vi "R3_Control.vi"() -> ()   [LabVIEW 2016]
uses:
  R3 Reactor Status v1.ctl
  R3 pH Manual Control.ctl
  R3 Pump Manual Control.ctl
  R3Variables.lvlib
panel:
  in  "SBR Timing":T1={"AR feeding"=0.0, "AR Decant"=0.0, "Anoxic feeding (min)"=90.0, "Anaerobic Time (min)"=110.0, "Anaerobic feeding (min)"=5.0, "Anoxic Time (min)"=0.0, "Aerobic Time (min) "=60.0, "Settle (min)"=20.0, "Decant (min)"=3.0}
  in  "R3 Pumps Manual Control":T2
  in  "Reactor 3 pH Control":T3
  out "R3 Reactor Status":T4 {"DO (mg/L)" format="%#_3g"; "pH" format="%#_3g"}
  out "Elapsed Time":dbl
  out "pH and DO":cluster{"pH":dbl, "DO (mg/L)":dbl}(graph)
  out "DO Intercept":dbl
  out "DO Slope":dbl
  out "pH Intercept":dbl
  out "pH Slope":dbl
  in  "pH Control":T5={" pH Set Point"=7.5, " pH Tolerance"=0.1, "Reaction Time (s)"=15.0, "Pump On Time (s)"=3.0}
  in  "Pumps Manual Control":bool
  in  "pH Manual Control":bool
  in  "DO Calibrate":bool
  in  "pH Calibrate":bool
  # "On: Manual Mode\nOff: SBR Mode"
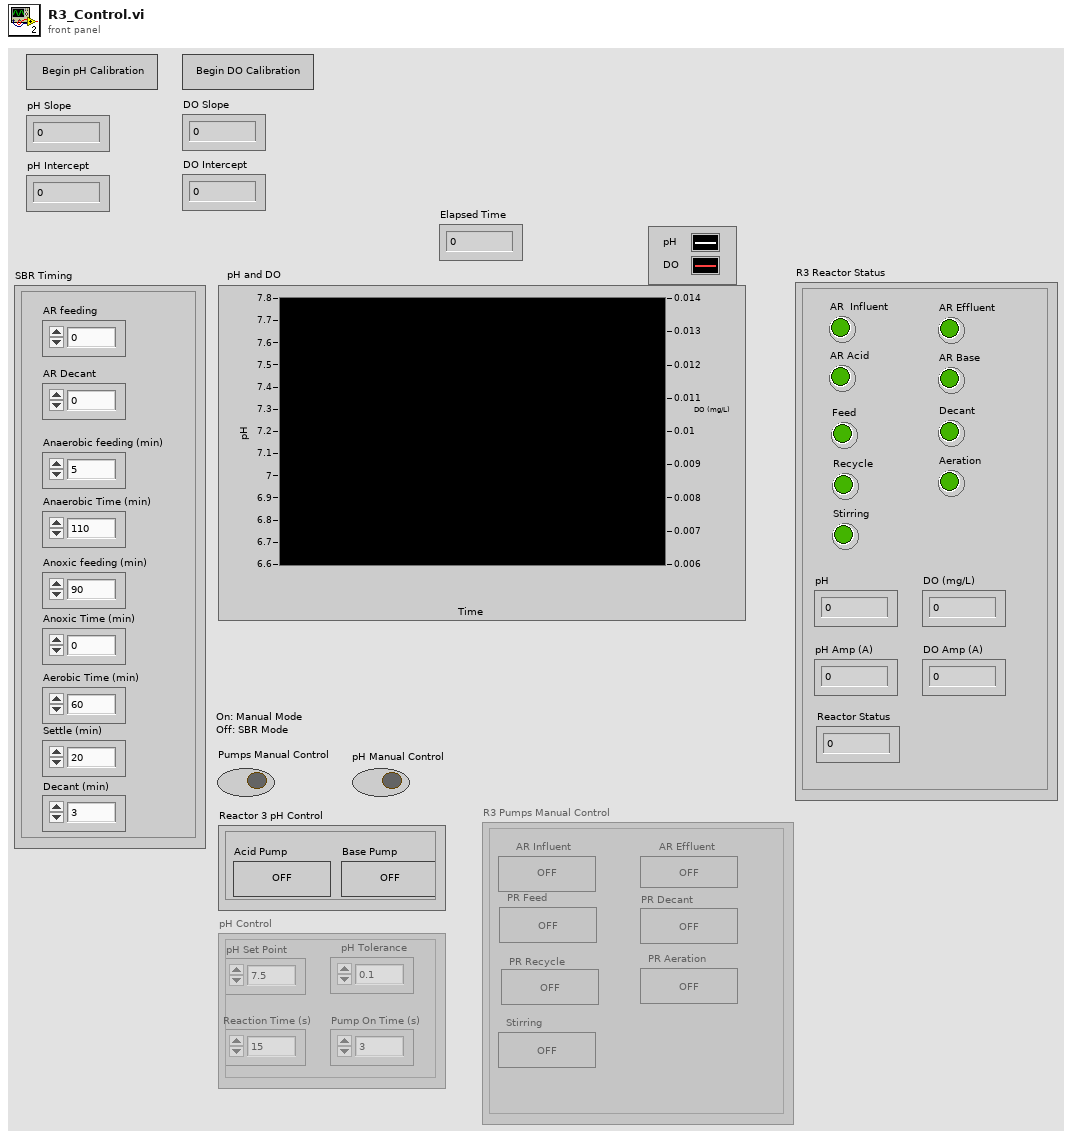
[diagram p1: front panel]
types:
  T1 = cluster{"AR feeding":dbl, "AR Decant":dbl, "Anoxic feeding (min)":dbl, "Anaerobic Time (min)":dbl, "Anaerobic feeding (min)":dbl, "Anoxic Time (min)":dbl, "Aerobic Time (min) ":dbl, "Settle (min)":dbl, "Decant (min)":dbl}
  T2 = cluster{"AR Influent":bool, "AR Effluent":bool, "PR Feed":bool, "PR Decant":bool, "PR Recycle":bool, "PR Aeration":bool, "Stirring":bool}
  T3 = typedef "R3Variables.lvlib/R3 pH Manual Control.ctl" = cluster{"Acid Pump":bool, "Base Pump":bool}
  T4 = typedef "R3Variables.lvlib/R3 Reactor Status v1.ctl" = cluster{"AR  Influent":bool, "AR Effluent":bool, "AR Acid":bool, "AR Base":bool, "Feed":bool, "Aeration":bool, "Decant":bool, "pH":dbl, "DO (mg/L)":dbl, "pH Amp (A)":dbl, "DO Amp (A)":dbl, "Recycle":bool, "Stirring":bool, "Reactor Status":dbl}
  T5 = cluster{" pH Set Point":dbl, " pH Tolerance":dbl, "Reaction Time (s)":dbl, "Pump On Time (s)":dbl}
  T6 = enum8{"Enabled", "Disabled", "Disabled and Grayed Out"}
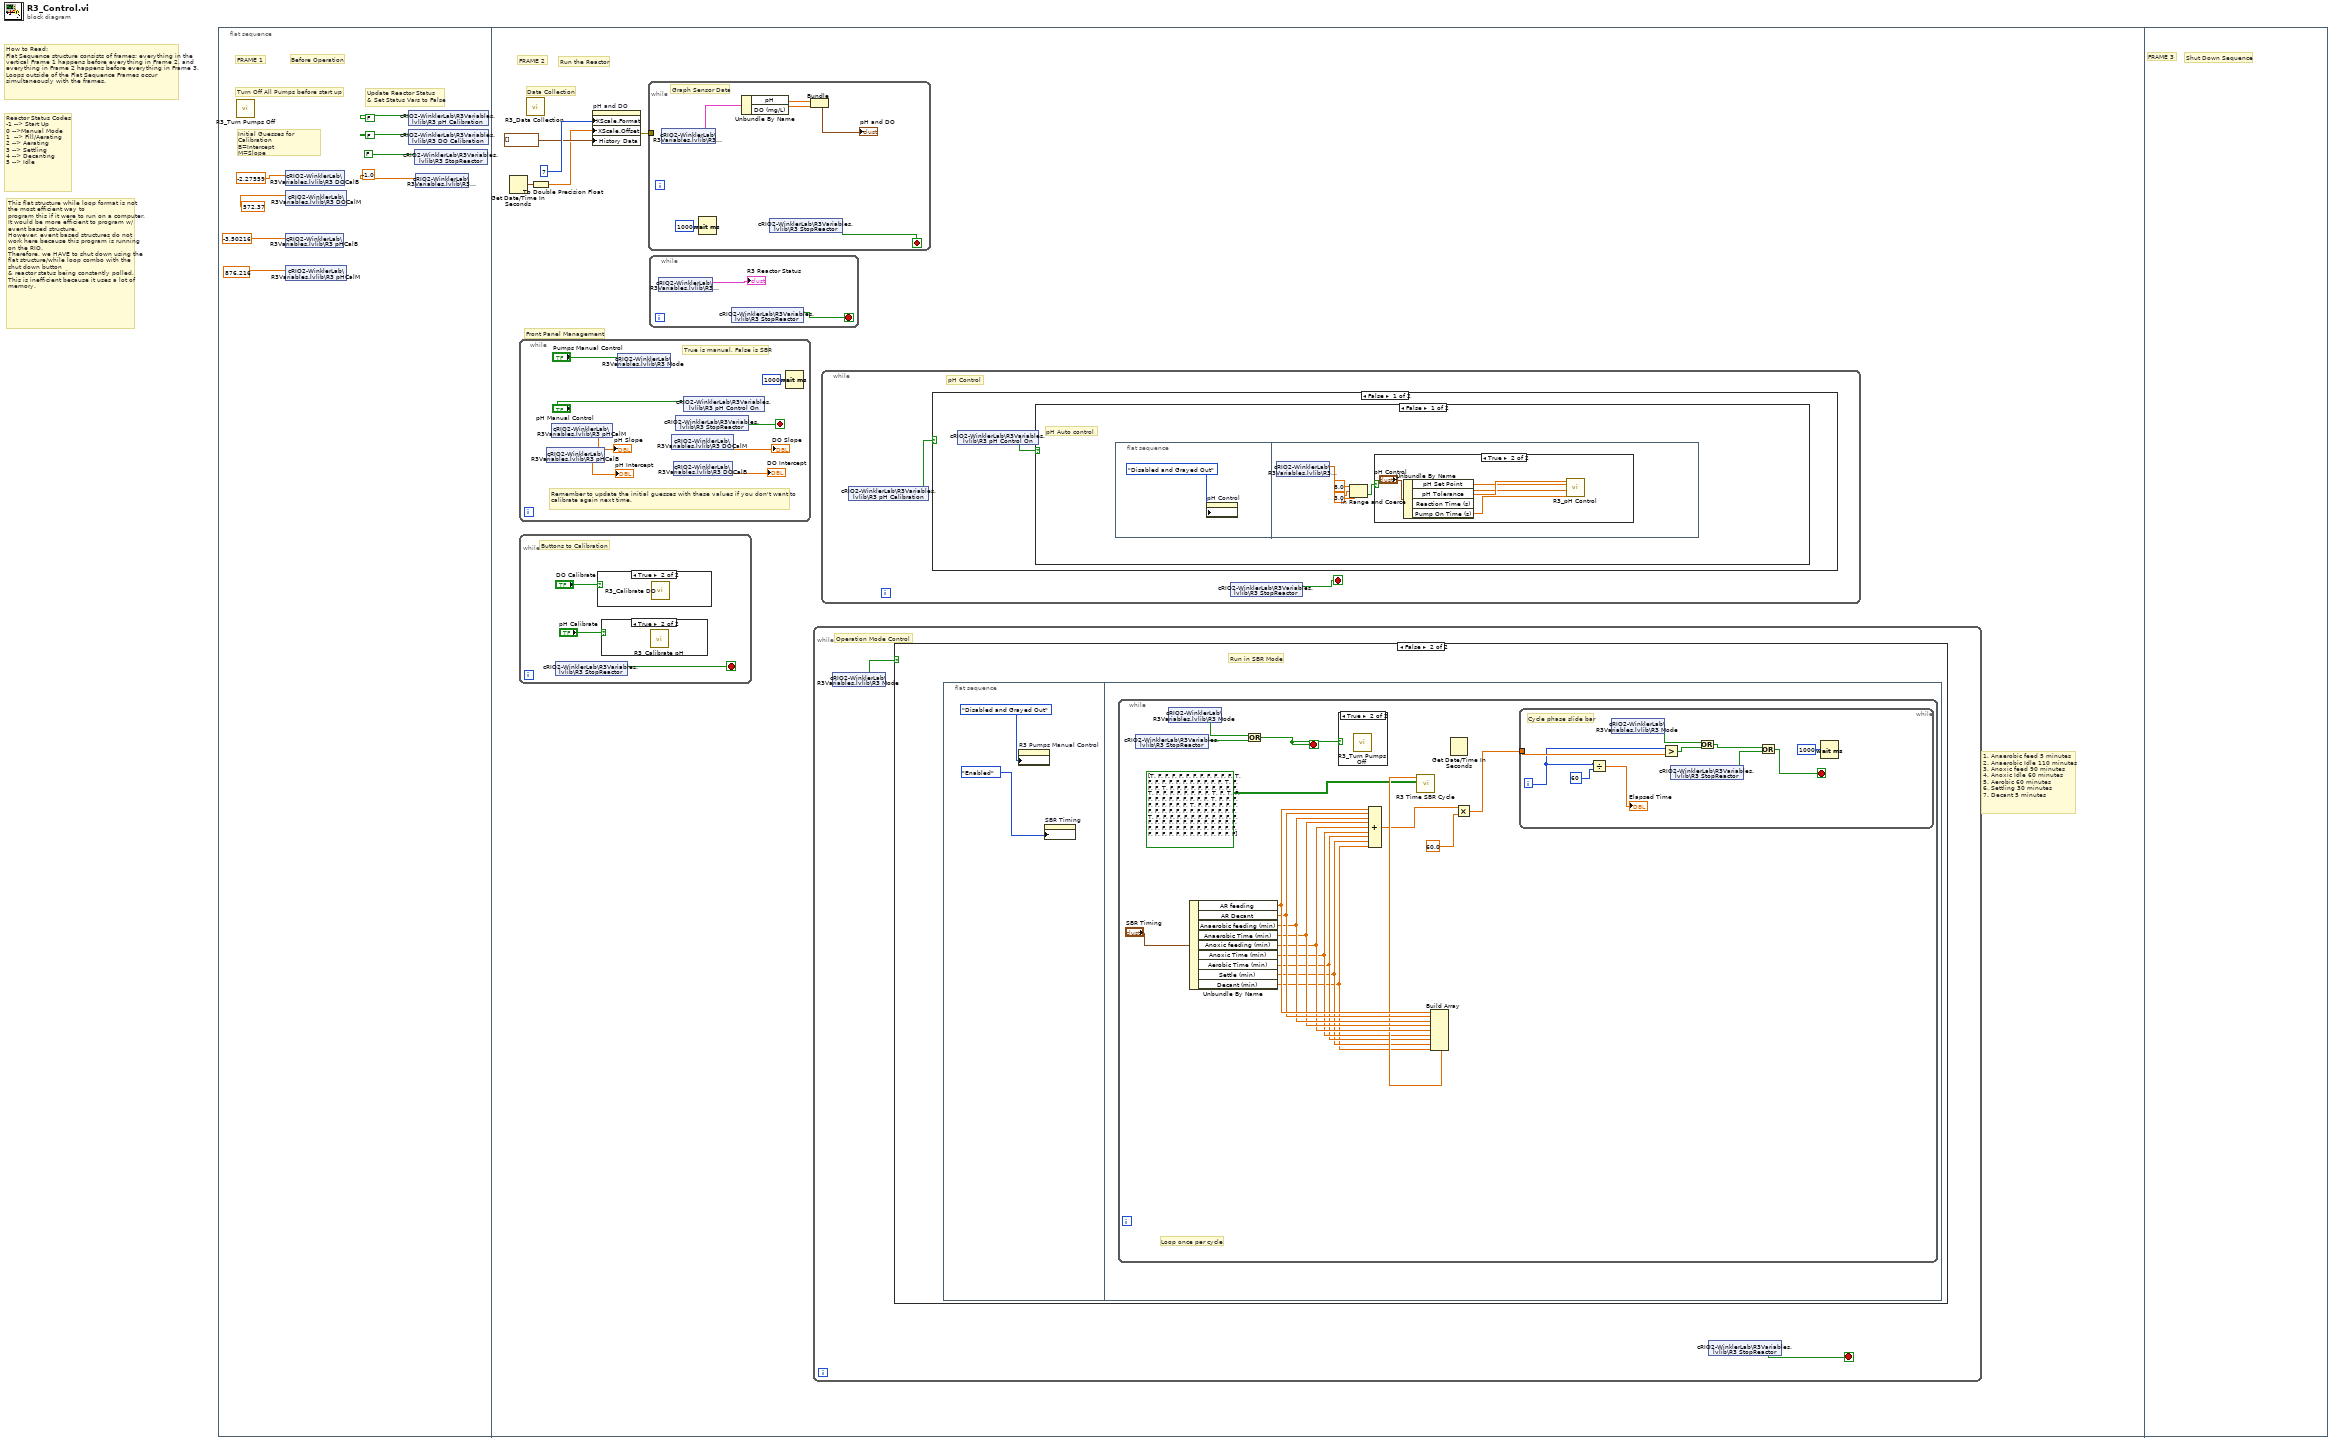
[diagram p0: block diagram]
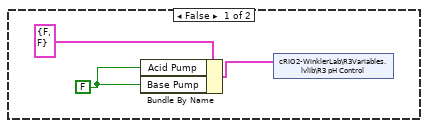
[diagram p4: hidden frame]
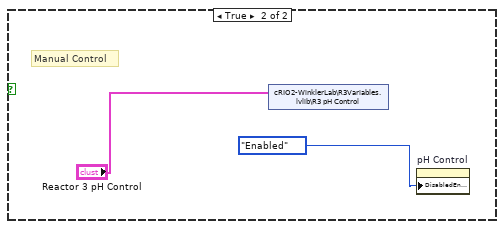
[diagram p5: hidden frame]
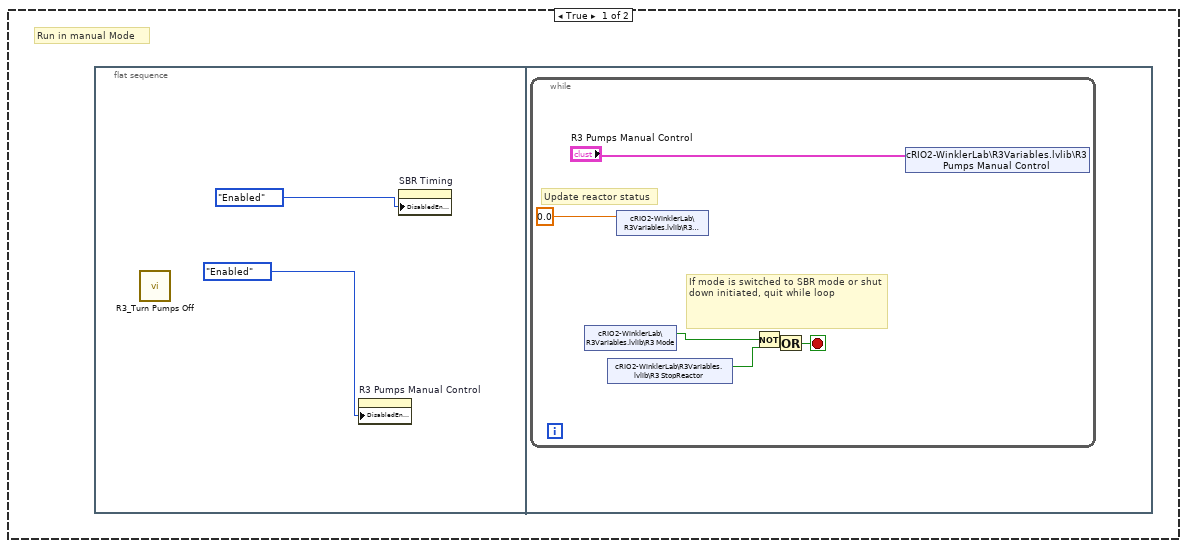
[diagram p7: hidden frame]
diagram:
  # "Reactor Status Codes\n-1 --> Start Up\n0 -->Manual Mode\n1  --> Fill/Aerating\n2 --> Aerating\n3 --> Settling\n4 --> Decanting\n5 --> Idle"
  # "How to Read:\nFlat Sequence structure consists of frames; everything in the vertical Frame 1 happens before everything in Frame 2, and everything in Frame 2 happens before everything in Frame 3.\nLoops outside of the Flat Sequence Frames occur simultaneously with the frames."
  # "This flat structure while loop format is not the most efficient way to \nprogram this if it were to run on a computer.\nIt would be more efficient to program w/ event based structure.\nHowever, event based structures do not work here because this program is running on the RIO.\nTherefore, we HAVE to shut down using the flat structure/while loop combo with the shut down button \n& reactor status being constantly polled.\nThis is inefficient because it uses a lot of memory."
  n1 = flat-sequence {
    frame #0 {
      # "Initial Guesses for Calibration\nB=Intercept\nM=Slope"
      # "Update Reactor Status \n& Set Status Vars to False"
      # "Turn Off All Pumps before start up"
      # "FRAME 1"
      # "Before Operation"
      n2 = call "R3_Turn Pumps Off.vi"() -> ()  [unwired: 12 in]
      n3 = shared-variable "cRIO2-WinklerLab\\R3Variables.lvlib\\R3 DOCalB"(-2.27559 ("R1DOxCalB")) -> ()  [unwired: 1 in, 1 out]
      n4 = shared-variable "cRIO2-WinklerLab\\R3Variables.lvlib\\R3 DOCalM"(572.37 ("R1DOxCalM")) -> ()  [unwired: 1 in, 1 out]
      n5 = shared-variable "cRIO2-WinklerLab\\R3Variables.lvlib\\R3 pHCalB"(-3.50216 ("R1pHCalB")) -> ()  [unwired: 1 in, 1 out]
      n6 = shared-variable "cRIO2-WinklerLab\\R3Variables.lvlib\\R3 pHCalM"(876.216 ("R1pHCalM")) -> ()  [unwired: 1 in, 1 out]
      n7 = shared-variable "cRIO2-WinklerLab\\R3Variables.lvlib\\R3 pH Calibration"(FALSE ("pH Calibration")) -> ()  [unwired: 1 in, 1 out]
      n8 = shared-variable "cRIO2-WinklerLab\\R3Variables.lvlib\\R3 DO Calibration"(FALSE ("DO Calibration")) -> ()  [unwired: 1 in, 1 out]
      n9 = shared-variable "cRIO2-WinklerLab\\R3Variables.lvlib\\R3 StopReactor"(FALSE ("R1Stop Reactor")) -> ()  [unwired: 1 in, 1 out]
      n10 = shared-variable "cRIO2-WinklerLab\\R3Variables.lvlib\\R3 Phase"(-1.0) -> ()  [unwired: 1 in, 1 out]
    }
    frame #1 {
      # "1. Anaerobic feed 5 minutes\n2. Anaerobic Idle 110 minutes \n3. Anoxic feed 90 minutes\n4. Anoxic Idle 60 minutes\n5. Aerobic 60 minutes\n6. Settling 30 minutes\n7. Decant 5 minutes"
      # "Front Panel Management"
      # "Data Collection"
      # "FRAME 2"
      # "Run the Reactor"
      n11 = Get Date/Time In Seconds() -> (seconds since 1Jan1904=w13:timestamp)
      n12 = while {
        stop <- w47 stop-if-true
        # "Remember to update the initial guesses with these values if you don't want to calibrate again next time."
        # "True is manual, False is SBR"
        n13 = shared-variable "cRIO2-WinklerLab\\R3Variables.lvlib\\R3 pHCalB"() -> (→"pH Intercept":dbl)  [unwired: 1 in, 1 out]
        n14 = shared-variable "cRIO2-WinklerLab\\R3Variables.lvlib\\R3 pHCalM"() -> (→"pH Slope":dbl)  [unwired: 1 in, 1 out]
        n15 = shared-variable "cRIO2-WinklerLab\\R3Variables.lvlib\\R3 Mode"("Pumps Manual Control") -> ()  [unwired: 1 in, 1 out]
        n16 = shared-variable "cRIO2-WinklerLab\\R3Variables.lvlib\\R3 DOCalM"() -> (→"DO Slope":dbl)  [unwired: 1 in, 1 out]
        n17 = shared-variable "cRIO2-WinklerLab\\R3Variables.lvlib\\R3 DOCalB"() -> (→"DO Intercept":dbl)  [unwired: 1 in, 1 out]
        n18 = shared-variable "cRIO2-WinklerLab\\R3Variables.lvlib\\R3 StopReactor"() -> (w47:bool)  [unwired: 1 in, 1 out]
        n19 = shared-variable "cRIO2-WinklerLab\\R3Variables.lvlib\\R3 pH Control On"("pH Manual Control") -> ()  [unwired: 1 in, 1 out]
        n20 = Wait (ms)(milliseconds to wait=u32 1000) -> ()  [unwired: 1 out]
      }
      n21 = while {
        stop <- w22 stop-if-true
        # "Buttons to Calibration"
        n22 = shared-variable "cRIO2-WinklerLab\\R3Variables.lvlib\\R3 StopReactor"() -> (w22:bool)  [unwired: 1 in, 1 out]
        n23 = case shown="True" "DO Calibrate" {
          frame False {
          }
          frame True {
            n24 = call "R3_Calibrate DO.vi"() -> ()  [unwired: 12 in]
          }
        }
        n25 = case shown="True" "pH Calibrate" {
          frame False {
          }
          frame True {
            n26 = call "R3_Calibrate pH.vi"() -> ()  [unwired: 12 in]
          }
        }
      }
      n27 = call "R3_Data Collection.vi"() -> ()  [unwired: 12 in]
      n28 = To Double Precision Float(number=w13) -> (double precision float=w9:dbl)
      n29 = property on="pH and DO" class="WFChart (strict)"("XScale.Format"=u8 7 ("X Scale.Display Format:Format"), "XScale.Offset"=w9, "History Data"=cluster{"pH":dbl, "DO (mg/L)":dbl}[] []) -> (error out=w12:errorcluster)  [unwired: 2 in, 1 out]
      n30 = while {
        tunnel: w12 -> [_]
        stop <- w18 stop-if-true
        # "Graph Sensor Data"
        n31 = shared-variable "cRIO2-WinklerLab\\R3Variables.lvlib\\R3 Status"() -> (w16:T4)  [unwired: 1 in, 1 out]
        n32 = Wait (ms)(milliseconds to wait=u32 1000) -> ()  [unwired: 1 out]
        n33 = Unbundle By Name(w16) -> ("pH"=w19:dbl, "DO (mg/L)"=w20:dbl)
        n34 = shared-variable "cRIO2-WinklerLab\\R3Variables.lvlib\\R3 StopReactor"() -> (w18:bool)  [unwired: 1 in, 1 out]
        n35 = Bundle("pH"=w19, "DO (mg/L)"=w20) -> (→"pH and DO":cluster{"pH":dbl, "DO (mg/L)":dbl})  [unwired: 1 in]
      }
      n36 = while {
        stop <- w15 stop-if-true
        n37 = shared-variable "cRIO2-WinklerLab\\R3Variables.lvlib\\R3 Status"() -> (→"R3 Reactor Status":T4)  [unwired: 1 in, 1 out]
        n38 = shared-variable "cRIO2-WinklerLab\\R3Variables.lvlib\\R3 StopReactor"() -> (w15:bool)  [unwired: 1 in, 1 out]
      }
      n39 = while {
        stop <- w52 stop-if-true
        # "Operation Mode Control"
        n40 = shared-variable "cRIO2-WinklerLab\\R3Variables.lvlib\\R3 Mode"() -> (w51:bool)  [unwired: 1 in, 1 out]
        n41 = case shown="False" w51 {
          frame True {
            # "Run in manual Mode"
            n42 = flat-sequence {
              frame #0 {
                n43 = call "R3_Turn Pumps Off.vi"() -> ()  [unwired: 12 in]
                n44 = property on="R3 Pumps Manual Control" class="Clust (strict)"("DisabledEnum"=T6."Enabled" ("Disabled")) -> ()  [unwired: 2 in, 2 out]
                n45 = property on="SBR Timing" class="Clust (strict)"("DisabledEnum"=T6."Enabled" ("Disabled")) -> ()  [unwired: 2 in, 2 out]
              }
              frame #1 {
                n46 = while {
                  stop <- w59 stop-if-true
                  # "If mode is switched to SBR mode or shut \ndown initiated, quit while loop"
                  # "Update reactor status"
                  n47 = shared-variable "cRIO2-WinklerLab\\R3Variables.lvlib\\R3 Mode"() -> (w57:bool)  [unwired: 1 in, 1 out]
                  n48 = shared-variable "cRIO2-WinklerLab\\R3Variables.lvlib\\R3 StopReactor"() -> (w56:bool)  [unwired: 1 in, 1 out]
                  n49 = shared-variable "cRIO2-WinklerLab\\R3Variables.lvlib\\R3 Phase"(0.0 ("Reactor Status")) -> ()  [unwired: 1 in, 1 out]
                  n50 = Not(x=w57) -> (.not. x?=w60:bool)
                  n51 = Or(x=w60, y=w56) -> (x .or. y?=w59:bool)
                  n52 = shared-variable "cRIO2-WinklerLab\\R3Variables.lvlib\\R3 Pumps Manual Control"("R3 Pumps Manual Control") -> ()  [unwired: 1 in, 1 out]
                }
              }
            }
          }
          frame False {
            # "Run in SBR Mode"
            n53 = flat-sequence {
              frame #0 {
                n54 = property on="R3 Pumps Manual Control" class="Clust (strict)"("DisabledEnum"=T6."Disabled and Grayed Out" ("Disabled")) -> ()  [unwired: 2 in, 2 out]
                n55 = property on="SBR Timing" class="Clust (strict)"("DisabledEnum"=T6."Enabled" ("Disabled")) -> ()  [unwired: 2 in, 2 out]
              }
              frame #1 {
                n56 = while {
                  stop <- w80 stop-if-true
                  # "Loop once per cycle"
                  n57 = shared-variable "cRIO2-WinklerLab\\R3Variables.lvlib\\R3 StopReactor"() -> (w78:bool)  [unwired: 1 in, 1 out]
                  n58 = shared-variable "cRIO2-WinklerLab\\R3Variables.lvlib\\R3 Mode"() -> (w79:bool)  [unwired: 1 in, 1 out]
                  n59 = Unbundle By Name("SBR Timing") -> ("AR feeding"=w77:dbl, "AR Decant"=w76:dbl, "Anaerobic feeding (min)"=w75:dbl, "Anaerobic Time (min)"=w74:dbl, "Anoxic feeding (min)"=w73:dbl, "Anoxic Time (min)"=w67:dbl, "Aerobic Time (min)"=w66:dbl, "Settle (min)"=w65:dbl, "Decant (min)"=w64:dbl)
                  n60 = Or(x=w79, y=w78) -> (x .or. y?=w80:bool)
                  n61 = case shown="True" w80 {
                    frame False {
                    }
                    frame True {
                      n62 = call "R3_Turn Pumps Off.vi"() -> ()  [unwired: 12 in]
                    }
                  }
                  n63 = Compound Arithmetic op=ADD(w77, w76, w75, w74, w73, w67, w66, w65, w64) -> (w68:dbl)
                  n64 = Build Array(w77, w76, w75, w74, w73, w67, w66, w65, w64) -> (w72:dbl[])
                  n65 = call "R3 Time SBR Cycle.vi"("Pump Status Array"=bool[][] [[TRUE, FALSE, FALSE, FALSE, FALSE, FALSE, FALSE, FALSE, FALSE, FALSE, FALSE], [FALSE, TRUE, FALSE, FALSE, FALSE, FALSE, FALSE, FALSE, FALSE, FALSE, FALSE], [FALSE, FALSE, TRUE, FALSE, FALSE, FALSE, TRUE, FALSE, FALSE, FALSE, FALSE], [FALSE, FALSE, FALSE, FALSE, FALSE, FALSE, TRUE, FALSE, FALSE, FALSE, FALSE], [FALSE, FALSE, FALSE, FALSE, TRUE, FALSE, TRUE, FALSE, FALSE, FALSE, FALSE], [FALSE, FALSE, FALSE, FALSE, FALSE, FALSE, TRUE, FALSE, FALSE, FALSE, FALSE], [FALSE, FALSE, FALSE, FALSE, FALSE, TRUE, FALSE, FALSE, FALSE, FALSE, FALSE], [FALSE, FALSE, FALSE, FALSE, FALSE, FALSE, FALSE, FALSE, FALSE, FALSE, FALSE], [FALSE, FALSE, FALSE, TRUE, FALSE, FALSE, FALSE, FALSE, FALSE, FALSE, FALSE], [FALSE, FALSE, FALSE, FALSE, FALSE, FALSE, FALSE, FALSE, FALSE, FALSE, FALSE], [FALSE, FALSE, FALSE, FALSE, FALSE, FALSE, FALSE, FALSE, FALSE, FALSE, FALSE], [FALSE, FALSE, FALSE, FALSE, FALSE, FALSE, FALSE, FALSE, FALSE, FALSE, FALSE], [FALSE, FALSE, FALSE, FALSE, FALSE, FALSE, FALSE, FALSE, FALSE, FALSE, FALSE]], "Timing Array"=w72) -> ()  [unwired: 10 in]
                  n66 = Get Date/Time In Seconds() -> ()  [unwired: 1 out]
                  n67 = Multiply(x=w68, y=60.0) -> (x*y=w69:dbl)
                  n68 = while {
                    tunnel: w69 -> [w89]
                    i -> [w83]
                    stop <- w84 stop-if-true
                    # "Cycle phase slide bar"
                    n69 = Divide(x=w83, y=60) -> (x/y=→"Elapsed Time":dbl)
                    n70 = shared-variable "cRIO2-WinklerLab\\R3Variables.lvlib\\R3 Mode"() -> (w86:bool)  [unwired: 1 in, 1 out]
                    n71 = Greater?(x=w83, y=w89) -> (0:w87:bool)
                    n72 = shared-variable "cRIO2-WinklerLab\\R3Variables.lvlib\\R3 StopReactor"() -> (w81:bool)  [unwired: 1 in, 1 out]
                    n73 = Or(x=w86, y=w87) -> (x .or. y?=w85:bool)
                    n74 = Or(x=w85, y=w81) -> (x .or. y?=w84:bool)
                    n75 = Wait (ms)(milliseconds to wait=u32 1000) -> ()  [unwired: 1 out]
                  }
                }
              }
            }
          }
        }
        n76 = shared-variable "cRIO2-WinklerLab\\R3Variables.lvlib\\R3 StopReactor"() -> (w52:bool)  [unwired: 1 in, 1 out]
      }
      n77 = while {
        stop <- w25 stop-if-true
        # "pH Control"
        n78 = shared-variable "cRIO2-WinklerLab\\R3Variables.lvlib\\R3 pH Calibration"() -> (w26:bool)  [unwired: 1 in, 1 out]
        n79 = case shown="False" w26 {
          frame False {
            n80 = shared-variable "cRIO2-WinklerLab\\R3Variables.lvlib\\R3 pH Control On"() -> (w27:bool)  [unwired: 1 in, 1 out]
            n81 = case shown="False" w27 {
              frame False {
                # "pH Auto control"
                n82 = flat-sequence {
                  frame #0 {
                    n83 = property on="pH Control" class="Clust (strict)"("DisabledEnum"=T6."Disabled and Grayed Out" ("Disabled")) -> ()  [unwired: 2 in, 2 out]
                  }
                  frame #1 {
                    n84 = shared-variable "cRIO2-WinklerLab\\R3Variables.lvlib\\R3 Phase"() -> (w31:dbl)  [unwired: 1 in, 1 out]
                    n85 = In Range and Coerce(upper limit=8.0, x=w31, lower limit=3.0) -> (In Range?=w29:bool)  [unwired: 1 out]
                    n86 = case shown="True" w29 {
                      frame False {
                        w35 = FALSE
                        n87 = Bundle By Name(cluster=T3 {"Acid Pump"=FALSE, "Base Pump"=FALSE} ("Reactor 3 pH Control"), "Acid Pump"=w35, "Base Pump"=w35) -> (w34:T3)
                        n88 = shared-variable "cRIO2-WinklerLab\\R3Variables.lvlib\\R3 pH Control"(w34) -> ()  [unwired: 1 in, 1 out]
                      }
                      frame True {
                        n89 = Unbundle By Name("pH Control") -> ("pH Set Point"=w38:dbl, "pH Tolerance"=w39:dbl, "Reaction Time (s)"=w37:dbl, "Pump On Time (s)"=w36:dbl)
                        n90 = call "R3_pH Control.vi"("Pump On Time (s)"=w36, "Reaction Time (s)"=w37, "pH Set Point"=w38, "pH Tolerance"=w39) -> ()  [unwired: 8 in]
                      }
                    }
                  }
                }
              }
              frame True {
                # "Manual Control"
                n91 = shared-variable "cRIO2-WinklerLab\\R3Variables.lvlib\\R3 pH Control"("Reactor 3 pH Control") -> ()  [unwired: 1 in, 1 out]
                n92 = property on="pH Control" class="Clust (strict)"("DisabledEnum"=T6."Enabled" ("Disabled")) -> ()  [unwired: 2 in, 2 out]
              }
            }
          }
          frame True {
          }
        }
        n93 = shared-variable "cRIO2-WinklerLab\\R3Variables.lvlib\\R3 StopReactor"() -> (w25:bool)  [unwired: 1 in, 1 out]
      }
    }
    frame #2 {
      # "FRAME 3"
      # "Shut Down Sequence"
    }
  }
